vi "VariantToType.vi"(11 "Variant":variant) -> (3 "type Name":string)   [LabVIEW 2015]
uses:
  <vilib>/Utility/VariantDataType/VariantType.lvlib
panel:
  # "Get Types of variant"
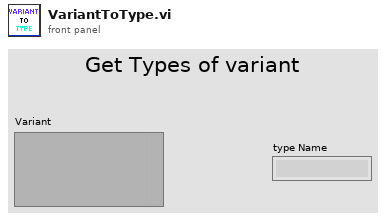
[diagram p1: front panel]
types:
  T1 = typedef "VariantType.lvlib/Type.ctl" = enum8{"Invalid Type", "Void", "I8", "I16", "I32", "I64", "U8", "U16", "U32", "U64", "Single Float", "Double Float", "Extended Float", "Single Complex", "Double Complex", "Extended Complex", "Enum U8", "Enum U16", "Enum U32", "Enum U64", "Single Float With Unit", "Double Float With Unit", "Extended Float With Unit", "Single Complex with Unit", "Double Complex with Unit", "Extended Complex with Unit", "Boolean", "String", "Path", "Picture", "Tag", "Array", "Cluster", "Variant", "LV Variant", "Waveform", "Timestamp", "Digital Waveform", "Digital Data", "ExpressData", "Refnum", "External Data", "VI", "Poly VI", "LabVIEW Class Instance", "Fixed Point"}
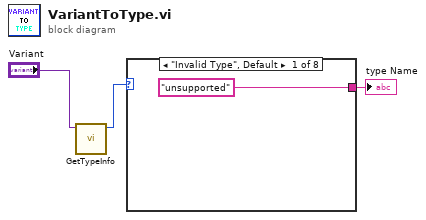
[diagram p0: block diagram]
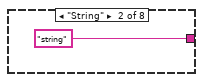
[diagram p2: hidden frame]
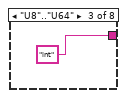
[diagram p3: hidden frame]
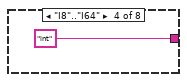
[diagram p4: hidden frame]
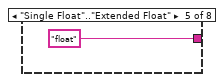
[diagram p5: hidden frame]
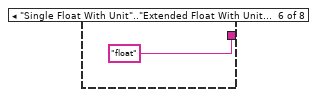
[diagram p6: hidden frame]
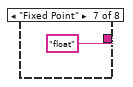
[diagram p7: hidden frame]
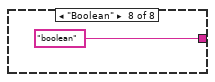
[diagram p8: hidden frame]
diagram:
  n1 = call <vilib>:"GetTypeInfo.vi"("Variant"="Variant") -> ("Type Enum"=w1:T1)  [unwired: 6 in, 4 out]
  n2 = case shown="\"Invalid Type\", Default" w1 {
    tunnel: ["unsupported" "string" "int" "int" "float" "float" "float" "boolean"] -> w3
    frame "Invalid Type", Default {
    }
    frame "String" {
    }
    frame "U8".."U64" {
    }
    frame "I8".."I64" {
    }
    frame "Single Float".."Extended Float" {
    }
    frame "Single Float With Unit".."Extended Float With Unit" {
    }
    frame "Fixed Point" {
    }
    frame "Boolean" {
    }
  }
  "type Name" <- w3
